vi "padé.vi"(1 "Retardo":dbl, 2 "Num\n Den":dbl[](array[numeric])) -> (0 "Salida":dbl[](array[numeric]))   [LabVIEW 2019]
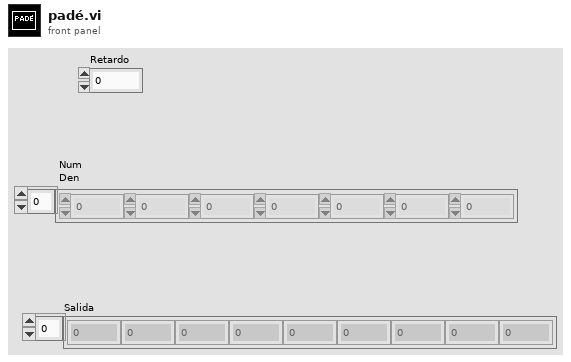
[diagram p1: front panel]
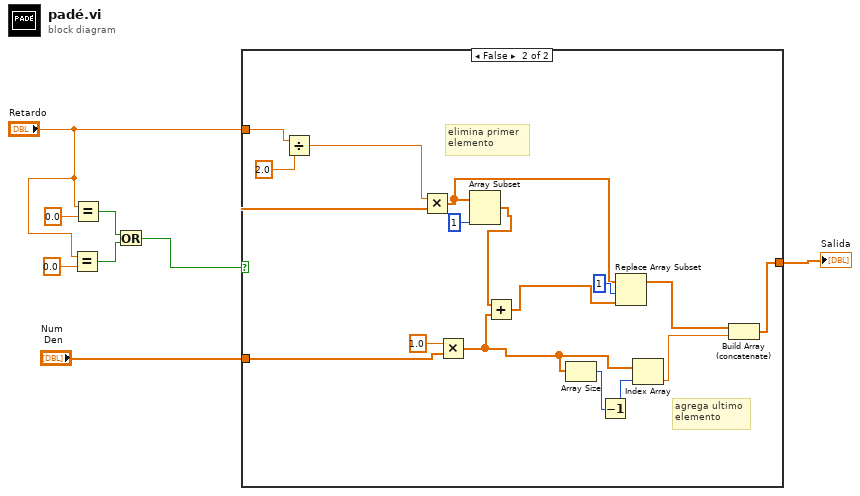
[diagram p0: block diagram]
diagram:
  n1 = Equal?(x="Retardo", y=0.0) -> (x = y?=w2:bool)
  n2 = Equal?(x="Retardo", y=0.0) -> (x = y?=w3:bool)
  n3 = Or(x=w3, y=w2) -> (x .or. y?=w1:bool)
  n4 = case shown="False" w1 {
    tunnel: [w9 w25] -> w8
    tunnel: "Num\n Den" -> [w9 w24]
    tunnel: "Retardo" -> [_ w10]
    frame True {
    }
    frame False {
      # "agrega ultimo\nelemento"
      # "elimina primer \nelemento"
      n5 = Divide(x=w10, y=2.0) -> (x/y=w11:dbl)
      n6 = Multiply(x=w11, y=w24) -> (x*y=w18:dbl[])
      n7 = Multiply(x=1.0, y=w24) -> (x*y=w17:dbl[])
      n8 = Array Subset(array=w18, index=1) -> (w21:dbl[])  [unwired: 1 in]
      n9 = Add(x=w21, y=w17) -> (x+y=w20:dbl[])
      n10 = Array Size(array=w17) -> (size(s)=w16:i32)
      n11 = Decrement(x=w16) -> (x-1=w15:i32)
      n12 = Replace Array Subset(array=w18, new element=w20, index=1) -> (w14:dbl[])
      n13 = Index Array(array=w17, index=w15) -> (element=w13:dbl)
      n14 = Build Array (concatenate)(w14, w13) -> (w25:dbl[])
    }
  }
  "Salida" <- w8
